vi "SoundEmission.vi"   [LabVIEW 2018]
doc: "Emette un suono"
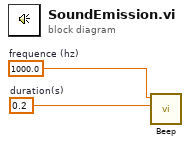
[diagram p0: block diagram]
diagram:
  w1 = 1000.0  # frequence (hz)
  w2 = 0.2  # duration(s)
  n1 = call <vilib>:"Beep.vi"("duration (msec) - ignored"=w2, "frequency (Hz) - ignored"=w1) -> ()  [unwired: 10 in]
